vi "FPGA Server.vi"() -> ()   [LabVIEW 2014]
doc: "Accepts inputs from a host based VI for controlling analog and digital outputs on a R-series board containing an FPGA. This VI will produce 4 different signal types dependent on the user input and the channel of interest. When the <B>WaveType</B> is set to laser, the first three channels will produce either a sine or square wave at the frequency <B>f0</B> while the last two produce only square waves. When the wavetype is set to speaker or none, all channels produce the same signal (although for the speaker, signals with a gain of <B>Amp</B> applied)."
uses:
  <vilib>/Platform/TimedLoop/XDataNode/timing_clust.ctl
  <vilib>/Platform/TimedLoop/XDataNode/nitl_modes.ctl
  <vilib>/Platform/TimedLoop/XDataNode/wakeup.ctl
  <vilib>/rvi/Emulation/niFpgaEmulationIsFPGAContextNoSignature.vi
  <vilib>/rvi/DataTransferAndStorage/Container/Common/niFpgaContainerGetUniqueNameForEmu.vi
  <vilib>/rvi/Memory/Memory_Emulation/niFpgaMemoryEmulationCacheClearOnFirstRun.vi
  <vilib>/rvi/Memory/Memory_Emulation/nirvimemoryEmulationManagerCache_MakeExclusive.vi
  <vilib>/rvi/Memory/Memory_Emulation/niFpgaMemoryEmulationValidateCache.vi
  <vilib>/rvi/Memory/Memory_Emulation/nirvimemoryEmulationManagerCache_InsertValue.vi
  <vilib>/Utility/error.llb/Clear Errors.vi
  <vilib>/rvi/Memory/Memory_Emulation/nirvimemoryEmulationManagerCache_ReleaseExclusive.vi
  <vilib>/rvi/Memory/Memory_Emulation/nirvimemoryEmulationManagerCache_GetValue.vi
  <vilib>/rvi/Memory/Memory_Emulation/nirvimemoryEmulationManagerCache_SetValue.vi
  <vilib>/rvi/Emulation/niFpgaProcessEmulError.vi
  <vilib>/rvi/Emulation/niFpgaSctlEmulationGetInTimedLoop.vi
  <vilib>/rvi/Emulation/niFpgaGetClockAttributes.vi
  <vilib>/rvi/Emulation/niFpgaEmulationReportErrorSimple.vi
  <vilib>/rvi/eio/common/nirviEmuTemplateMethod_errors.vi
  <vilib>/rvi/Emulation/niFpgaCriticalErrorInLSC.vi
  <vilib>/rvi/interface/RandomDataEmulation/niFpgaRandomDataHandleErrors.vi
  <vilib>/rvi/DataTransferAndStorage/Container/XNode/niFpgaContainer.xnode
  <vilib>/rvi/DataTransferAndStorage/Register/Emulation/niFpgaRegisterEmulation.vi
  <vilib>/eio/EIONode/EIONode.xnode
  <vilib>/rvi/interface/RandomDataEmulation/nirviRandomDataFpgaReadWriteTemplate.vi
  <vilib>/Platform/TimedLoop/XDataNode/XDataNode.xnode
  <vilib>/Platform/TimedLoop/XDataNode/XDNodeRunTimeDep.lvlib
panel:
  out "stopped":bool
  in  "iSpk Enable":T1={"Ch1"=TRUE, "Ch2"=TRUE, "Ch3"=TRUE, "Ch4"=TRUE, "Ch5"=TRUE}
  in  "Speaker":cluster{"Voltage":fxp<+,32,0>, "Offset":i16}
  in  "Spk Enable":bool
  in  "LaserEn":T1
  in  "Cell 5":T2 {"Offset" format="%#.6f"}
  in  "Cell 4":T2 {"Offset" format="%#.6f"}
  in  "Cell 3":T2 {"Offset" format="%#.6f"}
  in  "Cell 2":T2 {"f0" format="%#.6g"; "Offset" format="%#.6f"}
  in  "Cell 1":T2 {"f0" format="%.0g"; "Offset" format="%#.6f"}
  out "SquareOut":T3
  in  "stop":bool
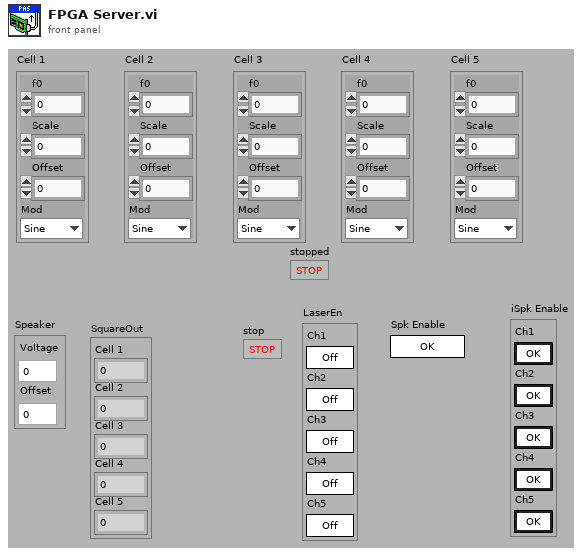
[diagram p1: front panel]
types:
  T1 = cluster{"Ch1":bool, "Ch2":bool, "Ch3":bool, "Ch4":bool, "Ch5":bool}
  T2 = cluster{"f0":fxp<+,32,0>, "Scale":fxp<+,32,0>, "Offset":i16, "Mod":enum8{"Sine", "Square"}}
  T3 = cluster{"Cell 1":i16, "Cell 2":i16, "Cell 3":i16, "Cell 4":i16, "Cell 5":i16}
  T4 = typedef "XDNodeRunTimeDep.lvlib/timing_clust.ctl" = cluster{"Expected End [f-1]":u64, "Actual End [f-1]":u64, "Finished Late? [f-1]":bool, "Expected End [i-1]":u64, "Actual End [i-1]":u64, "Finished Late? [i-1]":bool, "Expected Start [i]":u64, "Actual Start [i]":u64, "Expected Start [f]":u64, "Actual Start [f]":u64, "Source Name":string, "Structure Name":string, "Period":i64, "Deadline":i64, "Offset":i64, "Start":i64, "Priority":i32, "Timeout":i32, "Mode":T5, "Wakeup Reason":T6, "Error":errorcluster, "Source Type":string, "Secondary Source Type":string, "Global End Time":u64, "Global Start Time":u64, "Frame Duration":u64, "Iteration Duration":u64, "Assigned CPU":i32, "I/O Scan Engine Mode":u32}
  T5 = typedef "XDNodeRunTimeDep.lvlib/nitl_modes.ctl" = enum32{"No Change", "Process missed periods, maintain original phase", "Discard missed periods, maintain original phase", "Process missed periods, ignore original phase", "Discard missed periods, ignore original phase"}
  T6 = typedef "XDNodeRunTimeDep.lvlib/wakeup.ctl" = enum32{"Normal", "Aborted", "Asynchronous wakeup", "Timing source error", "Timed loop error", "Timeout"}
  T7 = cluster{"SW Out":i16, "SW Out":i16, "SW Out":i16, "SW Out":i16, "SW Out":i16}
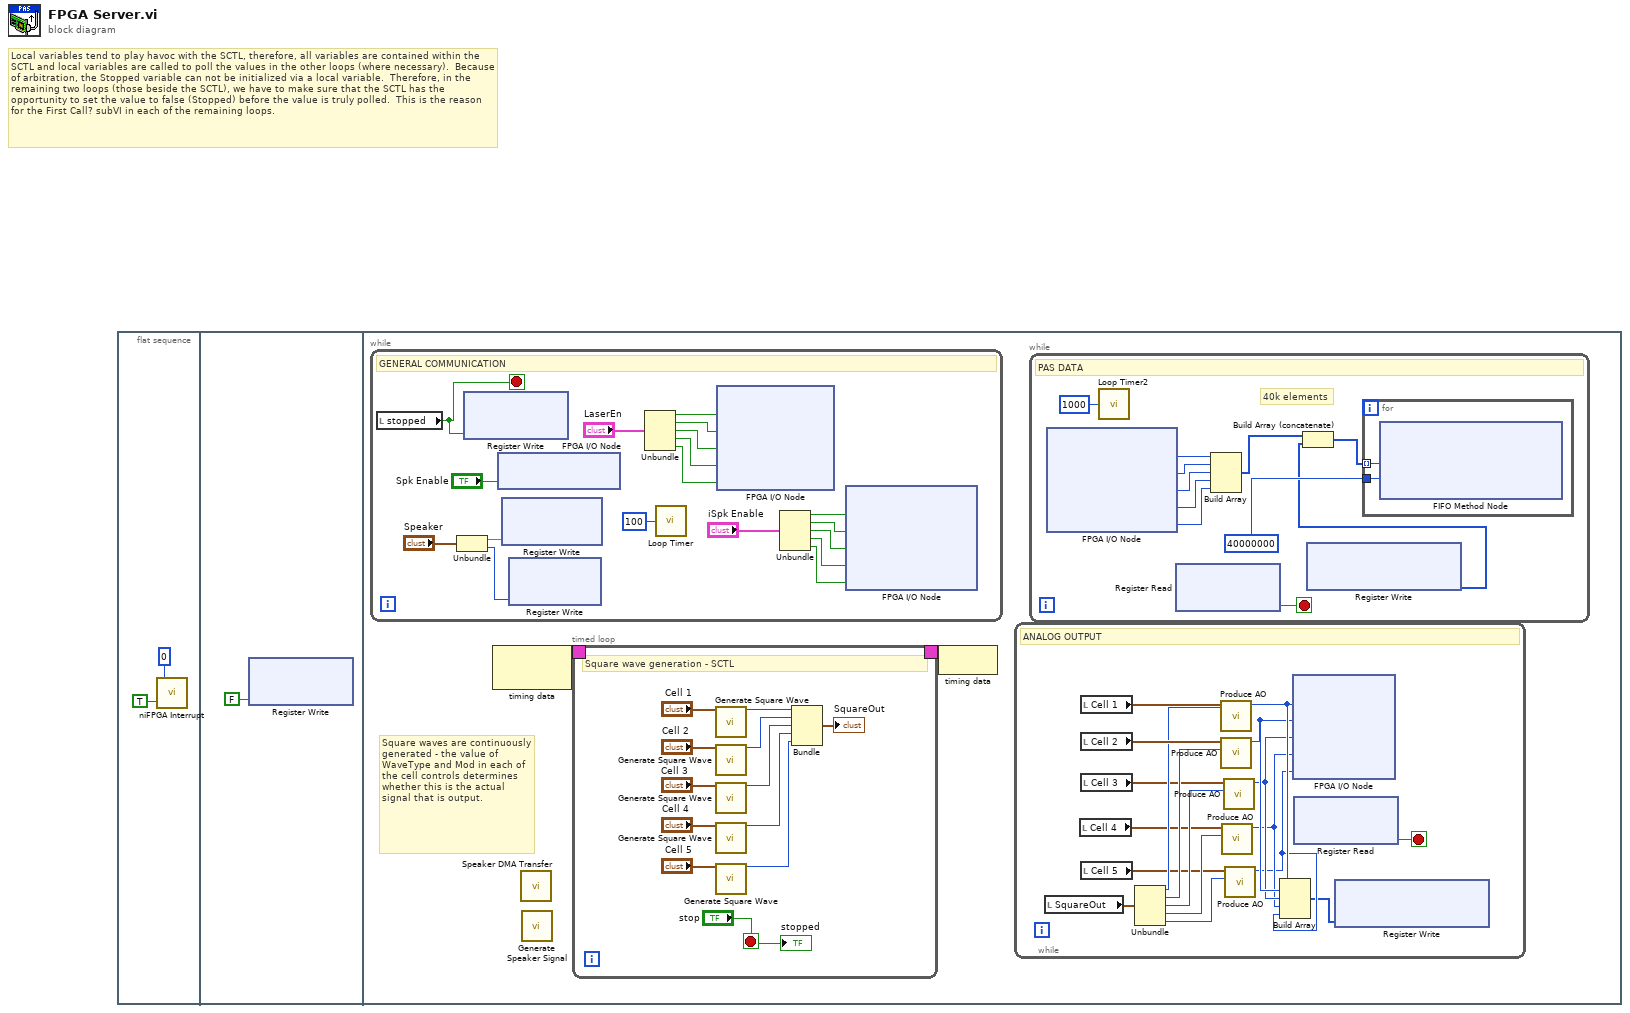
[diagram p0: block diagram]
diagram:
  # "Local variables tend to play havoc with the SCTL, therefore, all variables are contained within the SCTL and local variables are called to poll the values in the other loops (where necessary).  Because of arbitration, the Stopped variable can not be initialized via a local variable.  Therefore, in the remaining two loops (those beside the SCTL), we have to make sure that the SCTL has the opportunity to set the value to false (Stopped) before the value is truly polled.  This is the reason for the First Call? subVI in each of the remaining loops."
  n1 = flat-sequence {
    frame #0 {
      n2 = call <vilib>:"niFPGA Interrupt.vi"("Wait Until Cleared (F)"=TRUE, "IRQ Number (0)"=u8 0) -> ()  [unwired: 1 in]
    }
    frame #1 {
      n3 = xnode ("Register Write")("Data"=FALSE) -> ()  [unwired: 1 in, 1 out]
    }
    frame #2 {
      # "Square waves are continuously generated - the value of WaveType and Mod in each of the cell controls determines whether this is the actual signal that is output."
      n4 = while {
        stop <- w19 stop-if-true
        # "GENERAL COMMUNICATION"
        n5 = local read "stopped"() -> (w19:bool)
        n6 = Unbundle("Speaker") -> ("Voltage"=w20:fxp<+,32,0>, "Offset"=w21:i16)
        n7 = xnode ("Register Write")("Data"=w19) -> ()  [unwired: 1 in, 1 out]
        n8 = xnode "FPGA I/O Node"("Speaker Enable"="Spk Enable") -> ()  [unwired: 1 in, 1 out]
        n9 = xnode ("Register Write")("Data"=w20) -> ()  [unwired: 1 in, 1 out]
        n10 = xnode ("Register Write")("Data"=w21) -> ()  [unwired: 1 in, 1 out]
        n11 = Unbundle("LaserEn") -> ("Ch1"=w34:bool, "Ch2"=w33:bool, "Ch3"=w32:bool, "Ch4"=w31:bool, "Ch5"=w30:bool)
        n12 = call "Loop Timer"("Count(mSec)"=u32 100) -> ()  [unwired: 1 out]
        n13 = xnode "FPGA I/O Node"("Laser Enable 0"=w34, "Laser Enable 1"=w33, "Laser Enable 2"=w32, "Laser Enable 3"=w31, "Laser Enable 4"=w30) -> ()  [unwired: 5 in, 5 out]
        n14 = Unbundle("iSpk Enable") -> ("Ch1"=w29:bool, "Ch2"=w28:bool, "Ch3"=w27:bool, "Ch4"=w26:bool, "Ch5"=w25:bool)
        n15 = xnode "FPGA I/O Node"("Speaker Switch 0"=w29, "Speaker Switch 1"=w28, "Speaker Switch 2"=w27, "Speaker Switch 3"=w26, "Speaker Switch 4"=w25) -> ()  [unwired: 5 in, 5 out]
      }
      n16 = node-c288() -> (w5:T4)  [unwired: 1 in]
      n17 = call "Speaker DMA Transfer.vi"() -> ()  [unwired: 20 in]
      n18 = call "Generate Speaker Signal.vi"() -> ()  [unwired: 20 in]
      n19 = timed-loop "Square wave generation - SCTL" {
        timing: w5 -> [_]
        timing-out: [_] -> w4
        stop <- "stop" stop-if-true
        # "Square wave generation - SCTL"
        n20 = call "Generate Square Wave.vi"("Laser Control"="Cell 1") -> ("SW Out"=w66:i16)  [unwired: 18 in]
        n21 = call "Generate Square Wave.vi"("Laser Control"="Cell 2") -> ("SW Out"=w61:i16)  [unwired: 18 in]
        n22 = call "Generate Square Wave.vi"("Laser Control"="Cell 3") -> ("SW Out"=w59:i16)  [unwired: 18 in]
        n23 = call "Generate Square Wave.vi"("Laser Control"="Cell 4") -> ("SW Out"=w57:i16)  [unwired: 18 in]
        n24 = call "Generate Square Wave.vi"("Laser Control"="Cell 5") -> ("SW Out"=w55:i16)  [unwired: 18 in]
        n25 = Bundle("SW Out"=w66, "SW Out"=w61, "SW Out"=w59, "SW Out"=w57, "SW Out"=w55) -> (→"SquareOut":T7)  [unwired: 1 in]
        "stopped" <- "stop"
      }
      n26 = node-c288(w4) -> ()
      n27 = while "Analog Output" {
        stop <- w43 stop-if-true
        # "ANALOG OUTPUT"
        n28 = local read "SquareOut"() -> (w54:T3)
        n29 = local read "Cell 4"() -> (w47:T2)
        n30 = local read "Cell 1"() -> (w53:T2)
        n31 = local read "Cell 2"() -> (w52:T2)
        n32 = local read "Cell 3"() -> (w49:T2)
        n33 = local read "Cell 5"() -> (w45:T2)
        n34 = Unbundle(w54) -> ("Cell 1"=w51:i16, "Cell 2"=w50:i16, "Cell 3"=w48:i16, "Cell 4"=w46:i16, "Cell 5"=w44:i16)
        n35 = call "Produce AO.vi"("SW Signal"=w51, "Cell 1"=w53) -> ("AO"=w42:i16)  [unwired: 8 in]
        n36 = call "Produce AO.vi"("SW Signal"=w50, "Cell 1"=w52) -> ("AO"=w41:i16)  [unwired: 8 in]
        n37 = call "Produce AO.vi"("SW Signal"=w46, "Cell 1"=w47) -> ("AO"=w39:i16)  [unwired: 8 in]
        n38 = call "Produce AO.vi"("SW Signal"=w48, "Cell 1"=w49) -> ("AO"=w40:i16)  [unwired: 8 in]
        n39 = call "Produce AO.vi"("SW Signal"=w44, "Cell 1"=w45) -> ("AO"=w38:i16)  [unwired: 8 in]
        n40 = Build Array(w42, w41, w40, w39, w38) -> (w37:i16[])
        n41 = xnode "FPGA I/O Node"("Laser Out 0"=w42, "Laser Out 1"=w41, "Laser Out 2"=w40, "Laser Out 3"=w39, "Laser Out 4"=w38) -> ()  [unwired: 5 in, 5 out]
        n42 = xnode ("Register Read")() -> ("Data"=w43:bool)  [unwired: 1 in, 1 out]
        n43 = xnode "Register Write"("Data"=w37) -> ()  [unwired: 1 in, 1 out]
      }
      n44 = while {
        stop <- w16 stop-if-true
        # "40k elements"
        # "PAS DATA"
        n45 = xnode "FPGA I/O Node"() -> ("Microphone In 0"=w14:i16, "Microphone In 1"=w13:i16, "Microphone In 2"=w12:i16, "Microphone In 3"=w11:i16, "Microphone In 4"=w10:i16)  [unwired: 5 in, 5 out]
        n46 = call "Loop Timer2"("Count(Ticks)"=u32 1000 ("Count(mSec)")) -> ()  [unwired: 1 out]
        n47 = xnode ("Register Read")() -> ("Data"=w16:bool)  [unwired: 1 in, 1 out]
        n48 = Build Array(w14, w13, w12, w11, w10) -> (w9:i16[])
        n49 = xnode "Register Write"() -> ("Data"=w6:i16[])  [unwired: 1 in, 1 out]
        n50 = Build Array (concatenate)(w9, w6) -> (w7:i16[])
        n51 = for {
          tunnel: w7 -> [w18] mode=indexing
          tunnel: 40000000 ("Timeout") -> [w17]
          n52 = xnode ("FIFO Method Node")("Element"=w18, "Timeout"=w17) -> ()  [unwired: 1 in, 2 out]
        }
      }
    }
  }
